vi "Wärmepumpe.VorlauftemperaturHeizkreislauf.vi"(0 "Wärmepumpe in":refnum<data-value>, 4 "Rücklauftemperatur  Heizkreislauf[°C]":dbl, 5 "Error in":errorcluster) -> (14 "Wärmepumpe out":refnum<data-value>, 19 "Error out":errorcluster)   [LabVIEW 2016, in "Wärmepumpe.lvclass"]
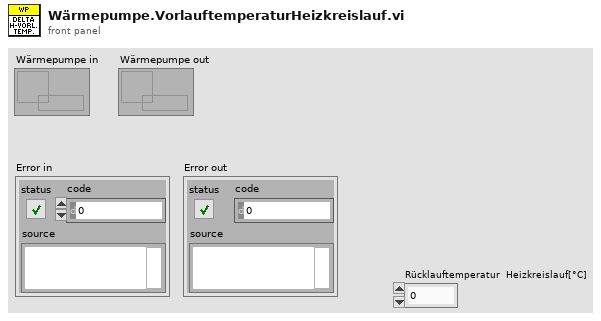
[diagram p1: front panel]
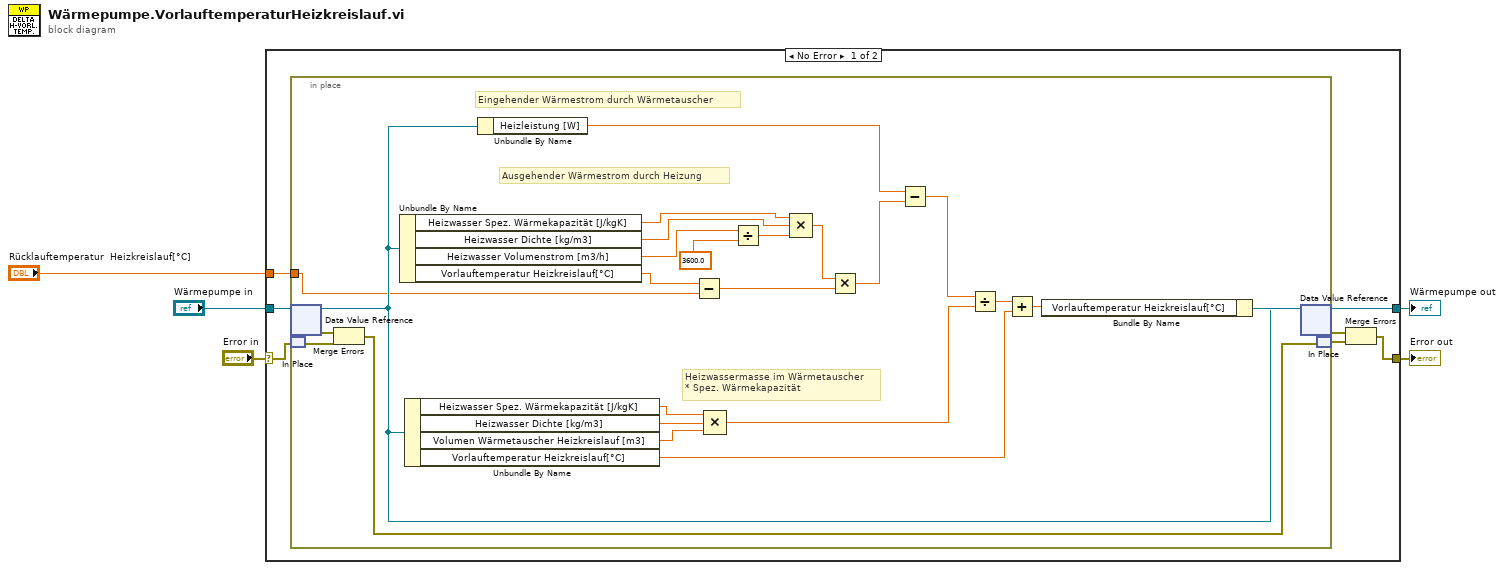
[diagram p0: block diagram]
diagram:
  n1 = case shown="No Error" "Error in" {
    selector: "Error in" -> [w10 w38]
    tunnel: [w9 w37] -> w3
    tunnel: [w8 w38] -> w2
    tunnel: "Wärmepumpe in" -> [w7 w37]
    tunnel: "Rücklauftemperatur  Heizkreislauf[°C]" -> [w6 _]
    frame No Error {
      n2 = in-place {
        in-place-border: w6 -> [w21]
        # "Heizwassermasse im Wärmetauscher\n* Spez. Wärmekapazität"
        # "Ausgehender Wärmestrom durch Heizung"
        # "Eingehender Wärmestrom durch Wärmetauscher"
        n3 = in-place-dvr #1(w7) -> (w27:refnum<class "Wärmepumpe.lvclass">, w36:errorcluster)
        n4 = in-place-match #2(w10) -> (w35:errorcluster)
        n5 = Merge Errors(w36, w35) -> (w34:errorcluster)
        n6 = Unbundle By Name(w27) -> ("Heizwasser Spez. Wärmekapazität [J/kgK]"=w16:dbl, "Heizwasser Dichte [kg/m3]"=w17:dbl, "Heizwasser Volumenstrom [m3/h]"=w18:dbl, "Vorlauftemperatur Heizkreislauf[°C]"=w22:dbl)
        n7 = Unbundle By Name(w27) -> ("Heizwasser Spez. Wärmekapazität [J/kgK]"=w14:dbl, "Heizwasser Dichte [kg/m3]"=w15:dbl, "Volumen Wärmetauscher Heizkreislauf [m3]"=w23:dbl, "Vorlauftemperatur Heizkreislauf[°C]"=w29:dbl)
        n8 = Unbundle By Name(w27) -> ("Heizleistung [W]"=w13:dbl)
        n9 = Subtract(x=w22, y=w21) -> (x-y=w25:dbl)
        n10 = Compound Arithmetic op=MULTIPLY(w14, w15, w23) -> (w28:dbl)
        n11 = Divide(x=w18, y=3600.0) -> (x/y=w19:dbl)
        n12 = Compound Arithmetic op=MULTIPLY(w16, w17, w19) -> (w26:dbl)
        n13 = Multiply(x=w26, y=w25) -> (x*y=w24:dbl)
        n14 = Subtract(x=w13, y=w24) -> (x-y=w33:dbl)
        n15 = Divide(x=w33, y=w28) -> (x/y=w32:dbl)
        n16 = Add(x=w32, y=w29) -> (x+y=w31:dbl)
        n17 = Bundle By Name(cluster=w27, "Vorlauftemperatur Heizkreislauf[°C]"=w31) -> (w30:refnum<class "Wärmepumpe.lvclass">)
        n18 = in-place-dvr #1(w30) -> (w9:refnum<data-value>, w12:errorcluster)
        n19 = in-place-match #2(w34) -> (w11:errorcluster)
      }
      n20 = Merge Errors(w12, w11) -> (w8:errorcluster)
    }
    frame Error {
    }
  }
  "Wärmepumpe out" <- w3
  "Error out" <- w2
